vi "Page_Info_Read.vi"(6 "ctlReferences":T1, 8 "error in (no error)":errorcluster, 11 "AB_DepDLL in":refnum<class "AB_DepDLL.lvclass">) -> (0 "error out":errorcluster, 3 "AB_DepDLL out":refnum<class "AB_DepDLL.lvclass">)   [LabVIEW 2020, in "AB_DepDLL.lvclass"]
uses:
  <vilib>/AppBuilder/AB_Classes/DepDLL/AB_DepDLL.lvclass
  e:/builds/penguin/labview/branches/2020/dev/dist/vi.lib/AppBuilder/AB_Classes/Build/AB_Build.lvclass
  <resource>/Framework/Providers/Builds/AppBuilder/AB_UI_Page_Info_References.ctl
  <vilib>/AppBuilder/AB_Classes/DLL/AB_DLL.lvclass
  <vilib>/AppBuilder/AB_Classes/Deployment/AB_Deployment.lvlib
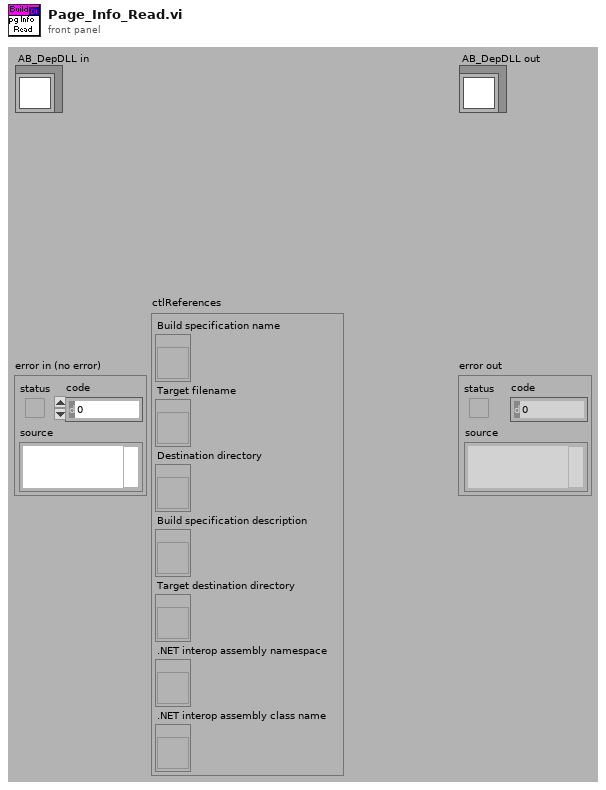
[diagram p1: front panel]
types:
  T1 = typedef "AB_UI_Page_Info_References.ctl" = cluster{"Build specification name":refnum<vi>, "Target filename":refnum<vi>, "Destination directory":refnum<vi>, "Build specification description":refnum<vi>, "Target destination directory":refnum<vi>, ".NET interop assembly namespace":refnum<vi>, ".NET interop assembly class name":refnum<vi>}
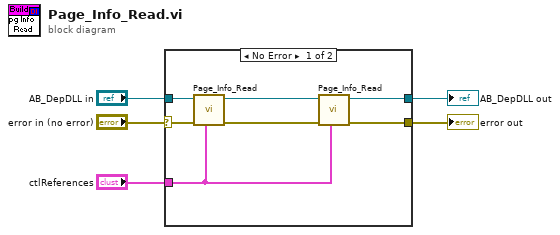
[diagram p0: block diagram]
diagram:
  n1 = case shown="No Error" "error in (no error)" {
    selector: "error in (no error)" -> [w12 w14]
    tunnel: [w7 w14] -> w2
    tunnel: "AB_DepDLL in" -> [w11 w13]
    tunnel: "ctlReferences" -> [w6 _]
    tunnel: [w9 w13] -> w1
    frame No Error {
      n2 = call-parent <vilib>:"Page_Info_Read.vi"("ctlReferences"=w6, "error in (no error)"=w12, "AB_Targetfile in"=w11) -> ("error out"=w8:errorcluster, "AB_Targetfile out"=w10:refnum<class "AB_DepDLL.lvclass">)  [unwired: 7 in]
      n3 = call <vilib>:"Page_Info_Read.vi"("ctlReferences"=w6, "error in (no error)"=w8, "Build in"=w10) -> ("error out"=w7:errorcluster, "Build out"=w9:refnum<class "AB_DepDLL.lvclass">)  [unwired: 7 in]
    }
    frame Error {
    }
  }
  "error out" <- w2
  "AB_DepDLL out" <- w1
